vi "GetAllItemsFromXMLFile.vi"() -> (3 "Array":refnum<class "Link.lvclass">[](array[class]))   [LabVIEW 2009, in "NavScreen.lvlib"]
uses:
  NavScreen.lvlib
  Classes/Link/Link.lvclass
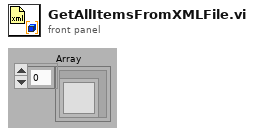
[diagram p1: front panel]
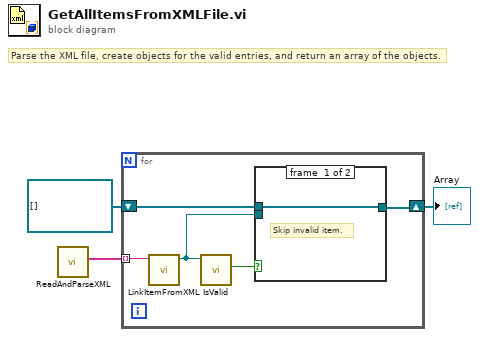
[diagram p0: block diagram]
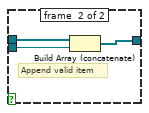
[diagram p2: hidden frame]
diagram:
  # "Parse the XML file, create objects for the valid entries, and return an array of the objects."
  n1 = call "ReadAndParseXML.vi"() -> ("XML Elements"=w3:string[])  [unwired: 11 in]
  n2 = for {
    tunnel: w3 -> [w8] mode=indexing
    shift-right: [w6] -> w2
    shift-left: refnum<class "Link.lvclass">[] [] -> [w7]
    n3 = call "LinkItemFromXML.vi"("XML for one item"=w8) -> ("GettingStartedWindow.lvlib:Link.lvclass"=w5:refnum<class "Link.lvclass">)  [unwired: 10 in]
    n4 = call "IsValid.vi"("Link in"=w5) -> ("valid"=w4:bool)  [unwired: 8 in, 2 out]
    n5 = case shown="True" w4 {
      tunnel: w7 -> [w9 w12]
      tunnel: [w9 w11] -> w6
      tunnel: w5 -> [_ w10]
      frame #0 {
        # "Skip invalid item."
      }
      frame #1 {
        # "Append valid item"
        n6 = Build Array (concatenate)(w12, w10) -> (w11:refnum<class "Link.lvclass">[])
      }
    }
  }
  "Array" <- w2
